vi "Get Image Data.vi"(7 "depth (24)":i32=24, 9 "subset rect":T1, 10 "Pic In":picture, 11 "Selection active?":bool) -> (2 "Pic Out":picture, 5 "image data out":T2={"image type"=0, "image depth"=24, "image"=array[3072 elements], "mask"=[255, 255, 255, 255, 128, 0, 0, 1, 128, 0, 0, 1, 128, 0, 0, 1, 128, 0, 0, 1, 128, 0, 0, 1, 128, 0, 0, 1, 128, 0, 0, 1, 128, 0, 0, 1, 128, 0, 0, 1, 128, 0, 0, 1, 128, 0, 0, 1, 128, 0, 0, 1, 128, 0, 0, 1, 128, 0, 0, 1, 128, 0, 0, 1, 128, 0, 0, 1, 128, 0, 0, 1, 128, 0, 0, 1, 128, 0, 0, 1, 128, 0, 0, 1, 128, 0, 0, 1, 128, 0, 0, 1, 128, 0, 0, 1, 128, 0, 0, 1, 128, 0, 0, 1, 128, 0, 0, 1, 128, 0, 0, 1, 128, 0, 0, 1, 128, 0, 0, 1, 128, 0, 0, 1, 255, 255, 255, 255], "colors"=[], "Rectangle"={"left"=0, "top"=0, "right"=32, "bottom"=32}})   [LabVIEW 2020, in "lv_icon.lvlib"]
doc: "Returns the Image Data Cluster."
uses:
  <vilib>/LabVIEW Icon API/lv_icon/lv_icon.lvlib
  <vilib>/picture/picture.llb/imagedata.ctl
  <vilib>/LabVIEW Icon API/LabVIEW Icon API.lvlib
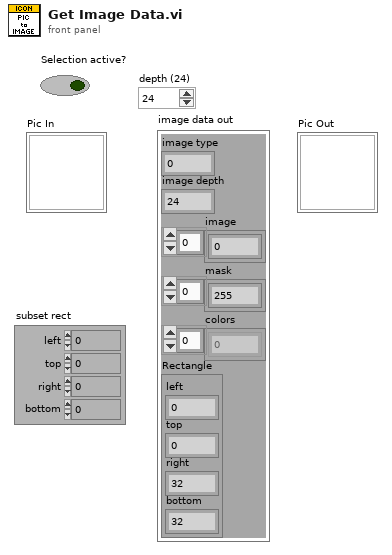
[diagram p1: front panel]
types:
  T1 = cluster{"left":i16, "top":i16, "right":i16, "bottom":i16}
  T2 = typedef "imagedata.ctl" = cluster{"image type":i32, "image depth":i32, "image":u8[], "mask":u8[], "colors":u32[], "Rectangle":cluster{"left":i16, "top":i16, "right":i16, "bottom":i16}}
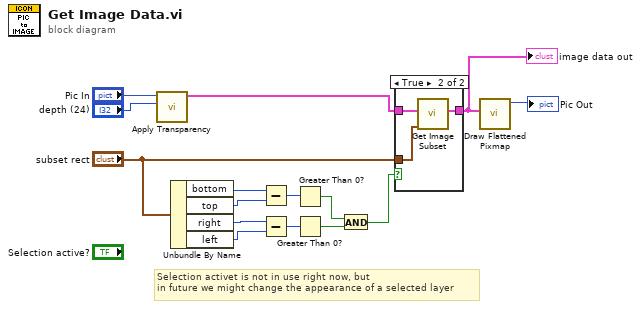
[diagram p0: block diagram]
diagram:
  # "Selection activet is not in use right now, but\nin future we might change the appearance of a selected layer"
  n1 = call <vilib>:"Apply Transparency.vi"("depth (24)"="depth (24)", "Pic In"="Pic In") -> ("image data"=w14:T2)  [unwired: 9 in]
  n2 = Unbundle By Name("subset rect") -> ("bottom"=w10:i16, "top"=w9:i16, "right"=w8:i16, "left"=w7:i16)
  n3 = Subtract(x=w10, y=w9) -> (x-y=w6:i16)
  n4 = Subtract(x=w8, y=w7) -> (x-y=w5:i16)
  n5 = Greater Than 0?(x=w6) -> (x > 0?=w3:bool)
  n6 = Greater Than 0?(x=w5) -> (x > 0?=w4:bool)
  n7 = And(x=w3, y=w4) -> (x .and. y?=w2:bool)
  n8 = case shown="True" w2 {
    tunnel: w14 -> [w16 w19]
    tunnel: [w16 w18] -> w13
    tunnel: "subset rect" -> [_ w17]
    frame False {
    }
    frame True {
      n9 = call <vilib>:"Get Image Subset.vi"("subset rect"=w17, "image data"=w19) -> ("image subset"=w18:T2)  [unwired: 5 out]
    }
  }
  "image data out" <- w13
  n10 = call <vilib>:"Draw Flattened Pixmap.vi"("image data"=w13) -> ("new picture"=→"Pic Out":picture)  [unwired: 1 in, 7 out]
